vi "Read Front Tunnels Refs.vi"(8 "error in (no error)":errorcluster, 11 "CSM-Helper in":refnum<class "CSM-Helper.lvclass">) -> (0 "error out":errorcluster, 2 "Front Tunnels":T1, 3 "CSM-Helper out":refnum<class "CSM-Helper.lvclass">)   [LabVIEW 2017, in "CSM-Helper.lvclass"]
doc: "### Read Front Tunnels Refs.vi\n\n-- <b>Controls</b> --\n- <b>CSM-Helper in</b>: CSMHelper input\n\n-- <b>Indicators</b> --\n- <b>Front Tunnels</b>:\n- <b>CSM-Helper out</b>: CSMHelper output"
uses:
  CSM-Helper.lvclass
  Typedef/_csmhelper_Front_Tunnels_Refs.ctl
  CSM-Helper.lvclass/CSM-Helper.ctl
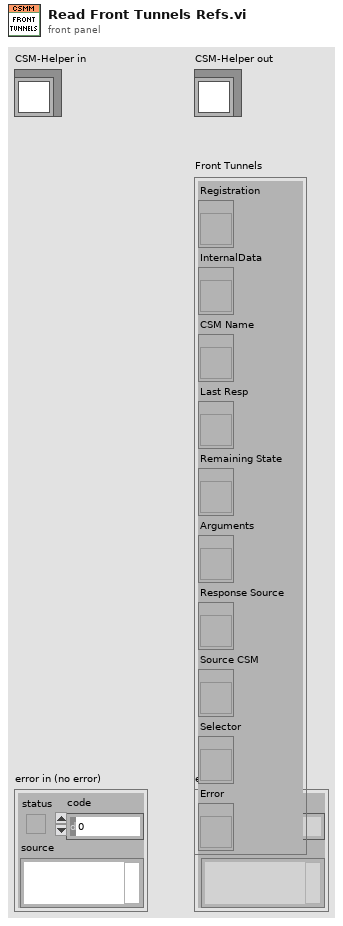
[diagram p1: front panel]
types:
  T1 = typedef "CSM-Helper.lvclass/_csmhelper_Front_Tunnels_Refs.ctl" = cluster{"Registration":refnum<vi>, "InternalData":refnum<vi>, "CSM Name":refnum<vi>, "Last Resp":refnum<vi>, "Remaining State":refnum<vi>, "Arguments":refnum<vi>, "Response Source":refnum<vi>, "Source CSM":refnum<vi>, "Selector":refnum<vi>, "Error":refnum<vi>}
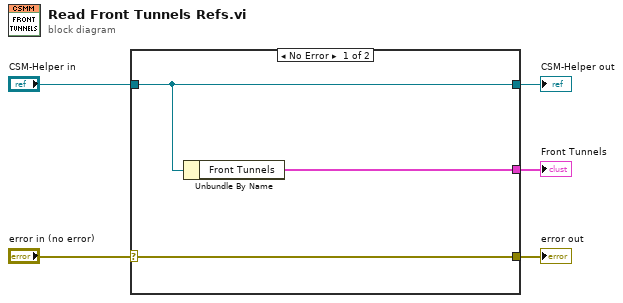
[diagram p0: block diagram]
diagram:
  n1 = case shown="No Error" "error in (no error)" {
    selector: "error in (no error)" -> [w8 w9]
    tunnel: [w8 w9] -> w4
    tunnel: [w7 w10] -> w2
    tunnel: "CSM-Helper in" -> [w7 w10]
    tunnel: [w6 _] -> w1
    frame No Error {
      n2 = Unbundle By Name(w7) -> ("Front Tunnels"=w6:T1)
    }
    frame Error {
    }
  }
  "error out" <- w4
  "CSM-Helper out" <- w2
  "Front Tunnels" <- w1
